vi "Demo.vi"() -> ()   [LabVIEW 2020, in "Tree Helpers.lvlib" / "Tag Tree.lvclass"]
uses:
  Tag Tree.lvclass
  Tag Tree.lvclass/Tag Tree.ctl
panel:
  out "Selected Tags":string[](array[string])
  in  "Tree":string[](tree)
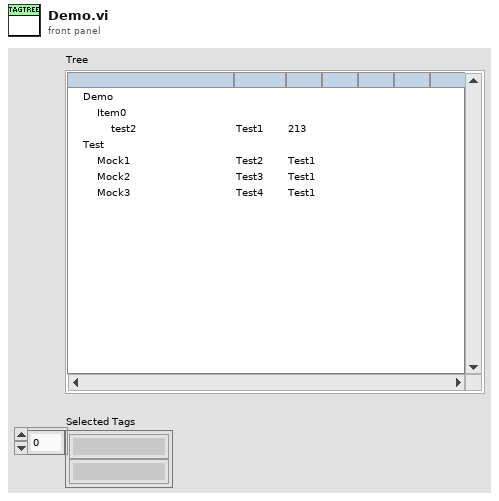
[diagram p1: front panel]
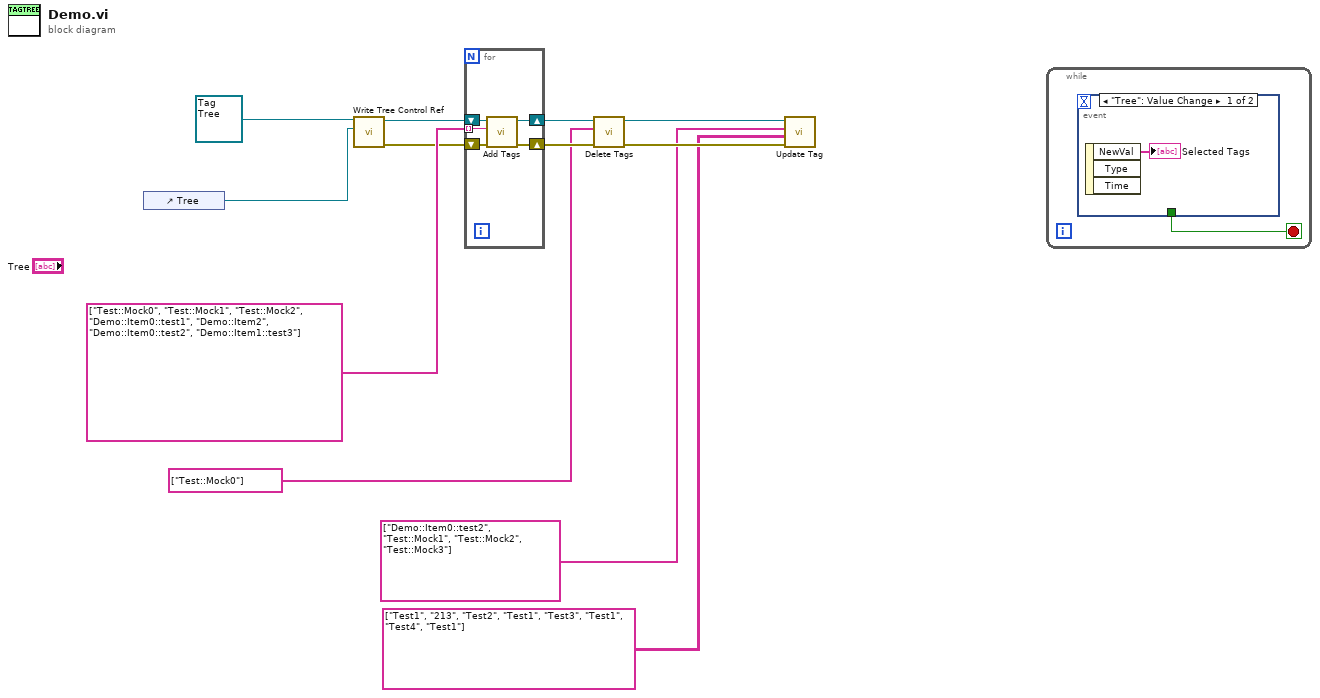
[diagram p0: block diagram]
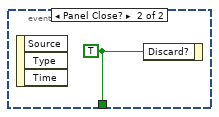
[diagram p2: hidden frame]
diagram:
  n1 = control-ref of="Tree"() -> (w11:refnum<vi>)
  n2 = call "Write Tree Control Ref.vi"("Tag Tree Reference"=w11, "Tag Tree In"=refnum<class "Tag Tree.lvclass"> refnum ("Support Utilities.lvlib:Tag Tree.lvclass")) -> ("error out"=w8:errorcluster, "Tag Tree Out"=w10:refnum<class "Tag Tree.lvclass">)  [unwired: 8 in]
  n3 = for {
    tunnel: string[] ["Test::Mock0", "Test::Mock1", "Test::Mock2", "Demo::Item0::test1", "Demo::Item2", "Demo::Item0::test2", "Demo::Item1::test3"] -> [w16] mode=indexing
    shift-right: [w14] -> w7
    shift-left: w10 -> [w17]
    shift-right: [w13] -> w6
    shift-left: w8 -> [w15]
    n4 = call "Add Tags.vi"("error in (no error)"=w15, "Tag"=w16, "Tag Tree In"=w17) -> ("error out"=w13:errorcluster, "Tag Tree Out"=w14:refnum<class "Tag Tree.lvclass">)  [unwired: 7 in]
  }
  n5 = call "Delete Tags.vi"("error in (no error)"=w6, "Tag"=string[] ["Test::Mock0"], "Tag Tree In"=w7) -> ("error out"=w4:errorcluster, "Tag Tree Out"=w3:refnum<class "Tag Tree.lvclass">)  [unwired: 7 in]
  n6 = call "Update Tag.vi"("error in (no error)"=w4, "Child Text"=string[][] [["Test1", "213"], ["Test2", "Test1"], ["Test3", "Test1"], ["Test4", "Test1"]], "Tag"=string[] ["Demo::Item0::test2", "Test::Mock1", "Test::Mock2", "Test::Mock3"], "Tag Tree In"=w3) -> ()  [unwired: 6 in, 2 out]
  n7 = while {
    stop <- w18 stop-if-true
    n8 = event shown="[0] \"Tree\": Value Change" {
      selector: _ -> [_ _]
      dyn-events: _ -> [_ _]
      timeout: _ -> [_ _]
      tunnel: [_ w20] -> w18
      event "Tree": Value Change {
        n9 = event-data() -> ("NewVal"=→"Selected Tags":string[])  [unwired: 1 in, 2 out]
      }
      event Panel Close? {
        w20 = TRUE ("Discard?")
        n10 = event-data() -> ()  [unwired: 1 in, 3 out]
        n11 = event-data ("Event Filter Node")("Discard?"=w20) -> ()  [unwired: 1 in, 1 out]
      }
    }
  }
